vi "Move Barre Splitter.vi"(8 "error in (no error)":errorcluster caption="entrée d'erreur (pas d'erreur)", 11 "UI Cam Basler en entrée":refnum<class "UI Cam Basler.lvclass">) -> (0 "error out":errorcluster caption="sortie d'erreur", 3 "UI Cam Basler en sortie":refnum<class "UI Cam Basler.lvclass">)   [LabVIEW 2023, in "UI Cam Basler.lvclass"]
uses:
  UI Cam Basler.lvclass
  UI Cam Basler.lvclass/UI Cam Basler.ctl
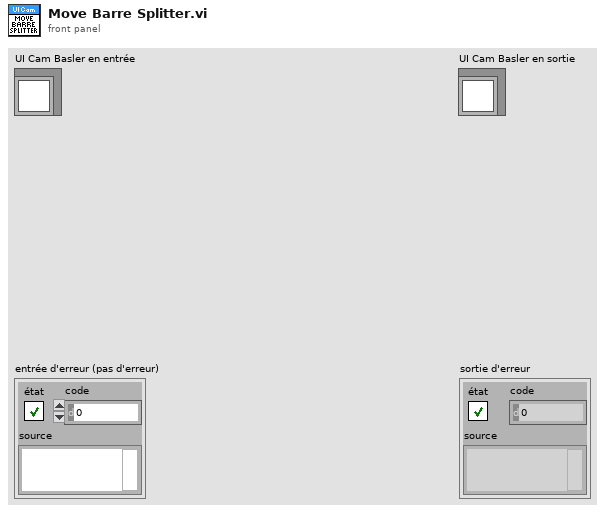
[diagram p1: front panel]
types:
  T1 = typedef "LVRectTypeDef.ctl" = cluster{"Left":i16, "Top":i16, "Right":i16, "Bottom":i16}
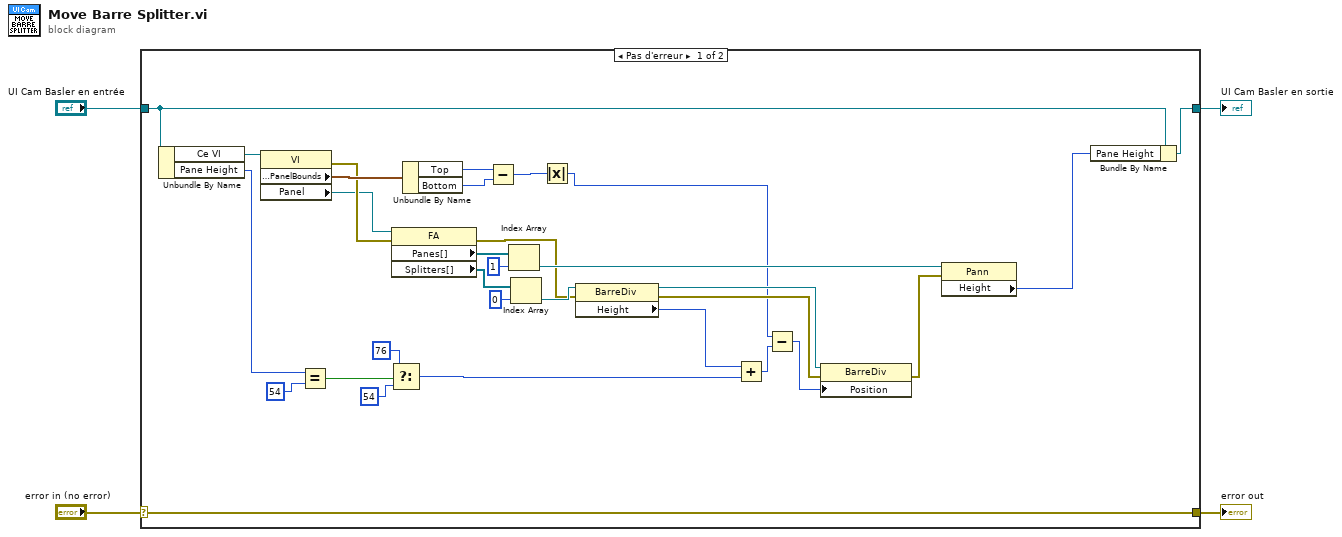
[diagram p0: block diagram]
diagram:
  n1 = case shown="Pas d'erreur" "error in (no error)" {
    selector: "error in (no error)" -> [w35 w37]
    tunnel: [w35 w37] -> w3
    tunnel: [w10 w36] -> w1
    tunnel: "UI Cam Basler en entrée" -> [w20 w36]
    frame No Error {
      n2 = Unbundle By Name(w20) -> ("Ce VI"=w19:refnum<vi>, "Pane Height"=w18:u32)
      n3 = property class="VI"(reference=w19) -> (error out=w30:errorcluster, "Front Panel.PanelBounds"=w31:T1, "Panel"=w29:refnum<vi>)  [unwired: 1 in, 1 out]
      n4 = Equal?(x=w18, y=u32 54) -> (x = y?=w15:bool)
      n5 = Select(t=u32 76 ("y"), s=w15, f=u32 54 ("y")) -> (s? t:f=w14:u32)
      n6 = property class="FA"(reference=w29, error in=w30) -> (error out=w22:errorcluster, "Panes[]"=w28:refnum<vi>[], "Splitters[]"=w25:refnum<vi>[])  [unwired: 1 out]
      n7 = Unbundle By Name(w31) -> ("Top"=w34:i16, "Bottom"=w33:i16)
      n8 = Subtract(x=w34, y=w33) -> (x-y=w32:i16)
      n9 = Index Array(array=w28, index=1 ("indice")) -> (element=w27:refnum<vi>)
      n10 = Index Array(array=w25, index=0 ("indice")) -> (element=w23:refnum<vi>)
      n11 = Absolute Value(x=w32) -> (abs(x)=w7:i16)
      n12 = property class="BarreDiv"(reference=w23, error in=w22) -> (reference out=w11:refnum<vi>, error out=w12:errorcluster, "Height"=w13:u32)
      n13 = Add(x=w13, y=w14) -> (x+y=w6:u32)
      n14 = Subtract(x=w7, y=w6) -> (x-y=w5:u32)
      n15 = property class="BarreDiv"(reference=w11, error in=w12, "Position"=w5) -> (error out=w9:errorcluster)  [unwired: 1 out]
      n16 = property class="Pann"(reference=w27, error in=w9) -> ("Height"=w8:u32)  [unwired: 2 out]
      n17 = Bundle By Name(cluster=w20, "Pane Height"=w8) -> (w10:refnum<class "UI Cam Basler.lvclass">)
    }
    frame Error {
    }
  }
  "error out" <- w3
  "UI Cam Basler en sortie" <- w1
